vi "Position find robot cancel Button.vi"(8 "Error In":errorcluster, 11 "Telem":refnum<vi>) -> (0 "Error Out":errorcluster)   [LabVIEW 2014]
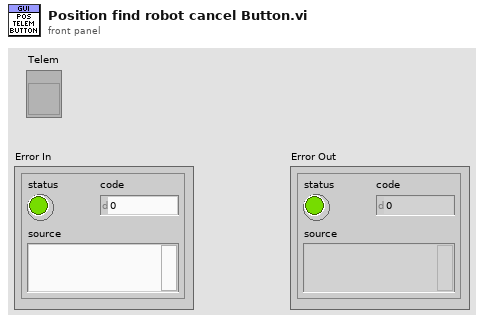
[diagram p1: front panel]
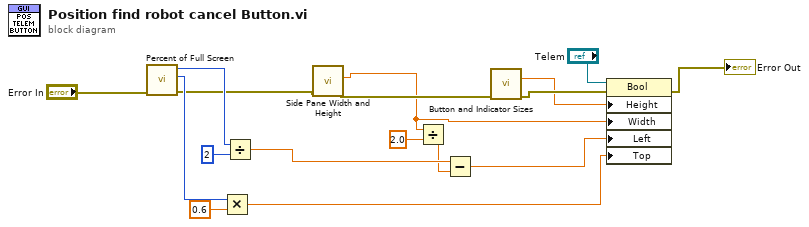
[diagram p0: block diagram]
diagram:
  n1 = call "Percent of Full Screen.vi"("error in (no error)"="Error In") -> ("error out"=w5:errorcluster, "Bottom"=w10:i16, "Right"=w15:i16)  [unwired: 8 in]
  n2 = Multiply(x=w10, y=0.6) -> (x*y=w8:dbl)
  n3 = Divide(x=w15, y=i16 2) -> (x/y=w13:dbl)
  n4 = call "Side Pane Width and Height.vi"("error in (no error)"=w5) -> ("error out"=w3:errorcluster, "Width"=w2:dbl)  [unwired: 8 in, 1 out]
  n5 = Divide(x=w2, y=2.0) -> (x/y=w12:dbl)
  n6 = Subtract(x=w13, y=w12) -> (x-y=w11:dbl)
  n7 = call "Button and Indicator Sizes.vi"("error in (no error)"=w3) -> ("Button Height"=w1:dbl, "error out"=w4:errorcluster)  [unwired: 10 in, 3 out]
  n8 = property class="Bool"(reference="Telem", error in=w4, "Height"=w1, "Width"=w2, "Left"=w11, "Top"=w8) -> (error out=→"Error Out":errorcluster)  [unwired: 1 out]
